vi "Ethernet_Reader.vi"(8 "에러 입력(에러 없음)":errorcluster, 10 "포트":u16=50, 11 "IP":string) -> (0 "에러 출력":errorcluster, 2 "R":u32, 3 "L":u32, 5 "Axis":string)   [LabVIEW 2014]
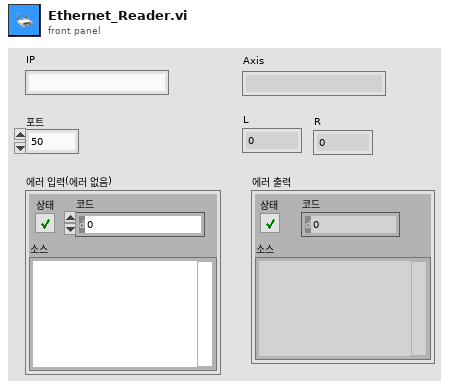
[diagram p1: front panel]
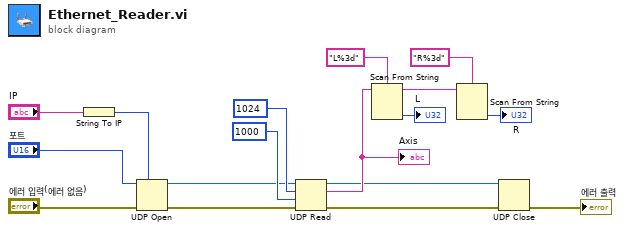
[diagram p0: block diagram]
diagram:
  n1 = String To IP(1:"IP") -> (0:w5:u32)
  n2 = UDP Open(7:w5, 8:"에러 입력(에러 없음)", 11:"포트") -> (port=w1:refnum<k16>, 0:w2:errorcluster)  [unwired: 2 in, 1 out]
  n3 = UDP Read(connection ID=w1, max size (548)=1024 ("최대 크기(548)"), timeout ms (25000)=1000 ("타임아웃 ms (25000)"), 8:w2) -> (data out=w15:string, error out=w9:errorcluster, 3:w8:refnum<k16>)  [unwired: 2 out]
  "Axis" <- w15
  n4 = Scan From String(format string="L%3d" ("포맷 문자열"), input string=w15) -> (remaining string=w14:string, output 1=→"L":u32)  [unwired: 3 in, 2 out]
  n5 = Scan From String(format string="R%3d" ("포맷 문자열"), input string=w14) -> (output 1=→"R":u32)  [unwired: 3 in, 3 out]
  n6 = UDP Close(connection ID=w8, 8:w9) -> (error out=→"에러 출력":errorcluster)  [unwired: 1 out]
